vi "Find_common_prefix.vi"(1 "Input Array":string[](array[string])) -> (0 "Common Characters":i32)   [LabVIEW 2020]
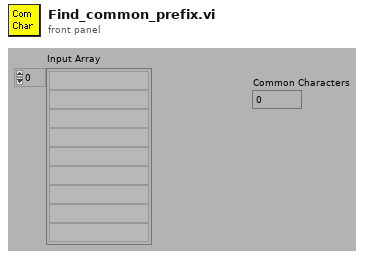
[diagram p1: front panel]
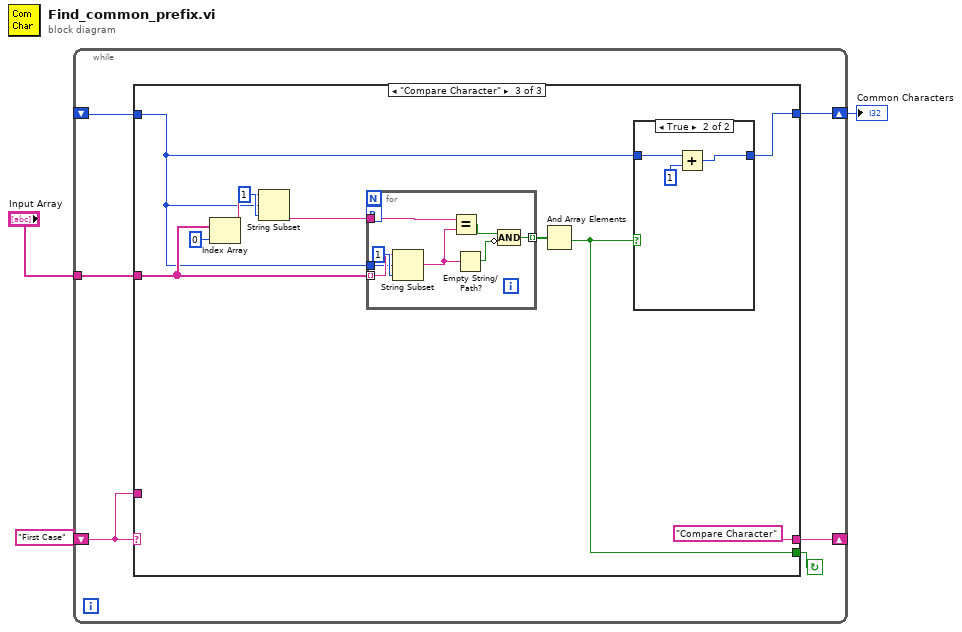
[diagram p0: block diagram]
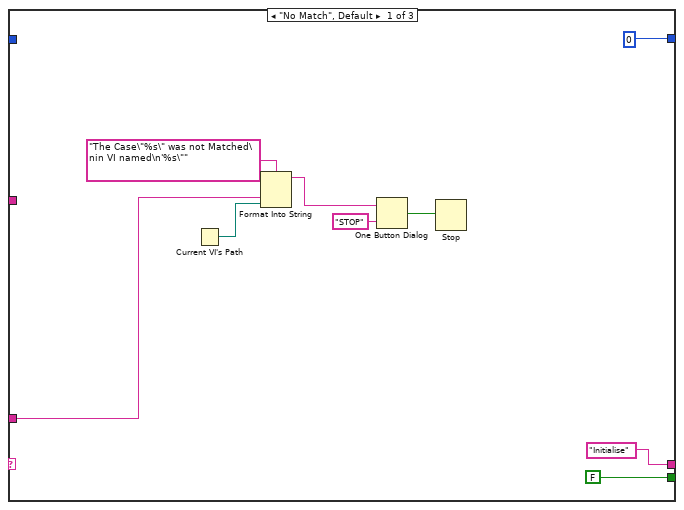
[diagram p2: hidden frame]
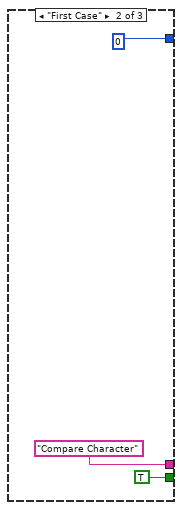
[diagram p3: hidden frame]
diagram:
  n1 = while {
    shift-left: _ -> [w4]
    shift-right: [w5] -> w1
    tunnel: "Input Array" -> [w6]
    shift-left: "First Case" -> [w7]
    shift-right: [w8] -> _
    stop <- w9 continue-if-true
    n2 = case shown="\"Compare Character\"" w7 {
      tunnel: [FALSE TRUE w22] -> w9
      tunnel: ["Initialise" "Compare Character" "Compare Character"] -> w8
      tunnel: w7 -> [w13 _ _]
      tunnel: w6 -> [_ _ w30]
      tunnel: [0 0 w24] -> w5
      tunnel: w4 -> [_ _ w25]
      frame "No Match", Default {
        n3 = Current VI's Path() -> (path=w12:path)
        n4 = Format Into String(format string="The Case\"%s\" was not Matched\nin VI named\n'%s\"" ("Format String"), w13, w12) -> (resulting string=w16:string)  [unwired: 2 in, 1 out]
        n5 = One Button Dialog(message=w16, button name ("OK")="STOP") -> (true=w14:bool)
        n6 = Stop(stop? (T)=w14) -> ()
      }
      frame "First Case" {
      }
      frame "Compare Character" {
        n7 = Index Array(array=w30, index=0 ("Index")) -> (element=w29:string)
        n8 = String Subset(string=w29, offset (0)=w25, length (rest)=1 ("length")) -> (substring=w27:string)
        n9 = for {
          tunnel: w30 -> [w42] mode=indexing
          tunnel: w25 -> [w41]
          tunnel: w27 -> [w39]
          tunnel: [w36] -> w26 mode=indexing
          workers-P: _ -> [_]
          n10 = String Subset(string=w42, offset (0)=w41, length (rest)=1 ("length")) -> (substring=w40:string)
          n11 = Equal?(x=w39, y=w40) -> (x = y?=w37:bool)
          n12 = Empty String/Path?(string/path=w40) -> (empty?=w38:bool)
          n13 = Compound Arithmetic op=AND(w37, invert w38) -> (w36:bool)
        }
        n14 = And Array Elements(Boolean array=w26) -> (logical AND=w22:bool)
        n15 = case shown="True" w22 {
          tunnel: w25 -> [w32 w35]
          tunnel: [w32 w34] -> w24
          frame False {
          }
          frame True {
            n16 = Add(x=w35, y=1) -> (x+y=w34:i32)
          }
        }
      }
    }
  }
  "Common Characters" <- w1
